vi "TranslucentBooleanProbe.vi"(1 "?":bool) -> (0 "Boolean":bool)   [LabVIEW 2017]
panel:
  out "Boolean value":bool
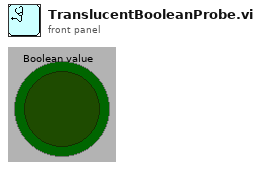
[diagram p1: front panel]
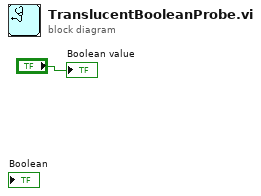
[diagram p0: block diagram]
diagram:
  "Boolean value" <- "?"
